vi "MU Write Register SSI.vi"(7 "values":u32[](array[numeric]), 8 "error in (no error)":errorcluster, 9 "count in":u32, 10 "address":u32, 11 "handle":u64) -> (0 "error out (no error)":errorcluster, 2 "count out":u32, 3 "function return":u32)   [LabVIEW 2017, in "MU_3SL_interface.lvlib"]
uses:
  MU_3SL_interface.lvlib
  lib/MU_3SL_interface.dll
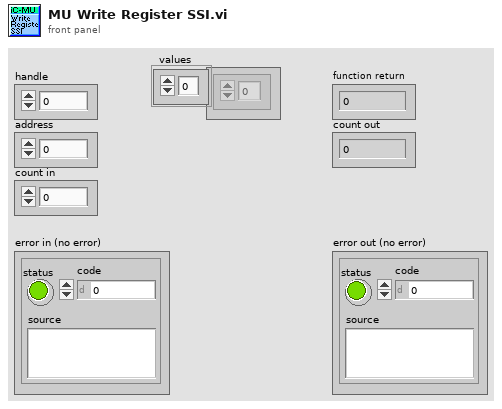
[diagram p1: front panel]
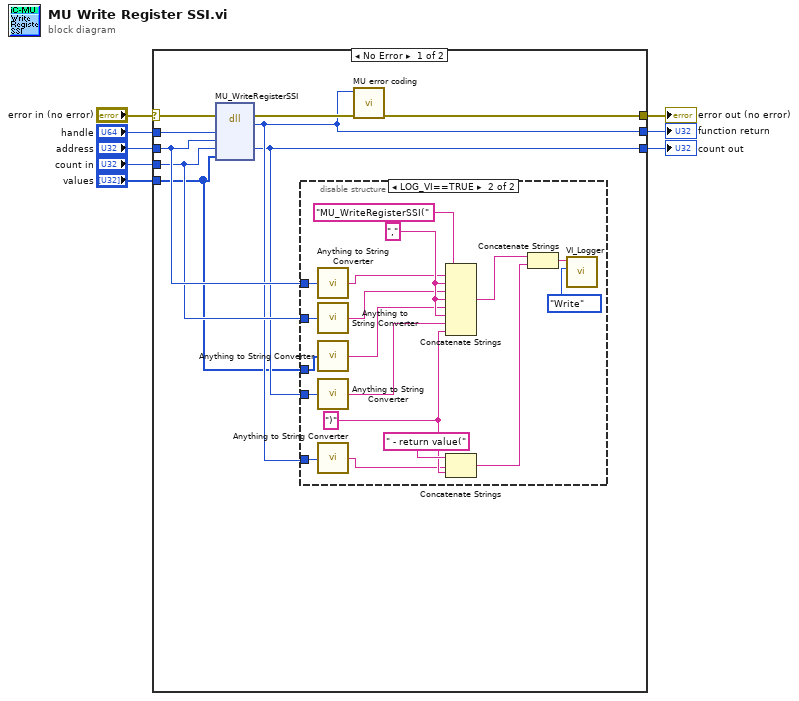
[diagram p0: block diagram]
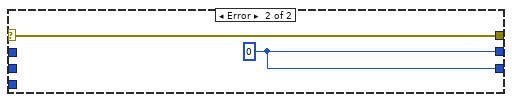
[diagram p3: hidden frame]
diagram:
  n1 = case shown="No Error" "error in (no error)" {
    selector: "error in (no error)" -> [w14 w37]
    tunnel: [w11 w36] -> w8
    tunnel: "handle" -> [w17 _]
    tunnel: "address" -> [w13 _]
    tunnel: "count in" -> [w12 _]
    tunnel: [w10 w36] -> w4
    tunnel: [w15 w37] -> w3
    tunnel: "values" -> [w9 _]
    frame No Error {
      n2 = dll-call lib="C:/Users/bes/AppData/Roaming/work/mu_9so/icsubmodules/soft_mu_3sl_master/lv_interface/lib/MU_3SL_interface**.*" fn="MU_WriteRegisterSSI"(error in=w14, "handle"=w17, "address"=w13, "count"=w12, "values"=w9) -> (error out=w16:errorcluster, "return type"=w11:u32, "count"=w10:u32)  [unwired: 5 in, 1 out]
      n3 = disable-structure shown="LOG_VI==TRUE" {
        disable-tunnel: w11 -> [_ w19]
        disable-tunnel: w13 -> [_ w27]
        disable-tunnel: w12 -> [_ w25]
        disable-tunnel: w10 -> [_ w22]
        disable-tunnel: w9 -> [_ w23]
        frame condition #0 {
        }
        frame condition #1 (active) {
          w29 = ")" ("string")
          w30 = "," ("string")
          n4 = call "Anything to String Converter.vi"("anything"=w27) -> ("String"=w26:string)
          n5 = call "Anything to String Converter.vi"("anything"=w25) -> ("String"=w24:string)
          n6 = call "Anything to String Converter.vi"("anything"=w23) -> ("String"=w21:string)
          n7 = call "Anything to String Converter.vi"("anything"=w22) -> ("String"=w20:string)
          n8 = call "Anything to String Converter.vi"("anything"=w19) -> ("String"=w18:string)
          n9 = Concatenate Strings("MU_WriteRegisterSSI(" ("Info in"), w26, w30, w24, w30, w21, w30, w20, w29) -> (w28:string)
          n10 = Concatenate Strings(" - return value(" ("string"), w18, w29) -> (w33:string)
          n11 = Concatenate Strings(w28, w33) -> (w32:string)
          n12 = call "VI_Logger.vi"("Action (Read)"=enum16{"Write", "Read"}."Write", "Info in"=w32) -> ()  [unwired: 8 in, 2 out]
        }
      }
      n13 = call "MU error coding.vi"("error in (no error)"=w16, "function return in"=w11) -> ("error out"=w15:errorcluster)  [unwired: 9 in]
    }
    frame Error {
      w36 = u32 0 ("return type")
    }
  }
  "function return" <- w8
  "count out" <- w4
  "error out (no error)" <- w3
